vi "Check_Settings_Case.vi"(6 "Queues":T1, 7 "Timer parameters":refnum<vi>, 8 "Status/Errors in":refnum<vi>, 9 "Control Parameters [] in":T2[](array[typedef]) {"Aux Byte Value" format="%02x"; "Max Real Value" format="%#_6e"; "Min Real Value" format="%#_6e"; "dReal/dByte" format="%#_6e"; "Byte Value" format="%02x"; "Identifier" format="%02x"}, 10 "Main parameters in":T5={"Mode"={"Mode"=enum."Dialog", "Expert?"=FALSE, "Dialog?"=FALSE}, "Stop loop"={"Settings changed?"=FALSE, "Stop?"=refnum}, "Send message"={"Send mode"=enum."Get parameters", "Set parameter list"=0, "Get parameter list"=0, "Reset device"=0, "Length set settings message"=0, "Reset buttons?"=FALSE, "Reset Master?"=enum."General"}, "Write settings"={"Options"=enum."File 1"}, "Settings state"={"MAS locked?"=refnum, "SLV locked?"=refnum}, "Button refs"={"Stop program"=refnum, "Save settings"=refnum, "DAQ mode"=refnum, "Reset settings"=refnum, "Apply settings"=refnum, "Reset MAS"=refnum, "Reset SLV"=refnum, "Local DBase?"=refnum, "Last value DBase"=FALSE, "Database"=refnum, "Calibration"=refnum, "Save settings 2"=refnum}, "Update screen"={"Detector number"=0, "Hardware"=enum."None"}, "Files"={"Path config file"=path "", "Path def. ini file"=path "", "Path ini file 1"=path "", "Path ini file 2"=path "", "Path RBF file"=path ""}, "DB connection"={"connection reference"=refnum, "Connected?"=refnum, "ODBC Name"=""}, "Status_id"=refnum, "Time difference"=refnum, "Satellites"=refnum, "Alignment parameters"=refnum, "Page Statistics 2"=refnum, "Database"=refnum, "Page Statistics"=refnum} {"Update screen"."Detector number" format="%#.0f"; "Send message"."Reset device" format="%x"; "Send message"."Get parameter list" format="%x"; "Send message"."Set parameter list" format="%x"}, 11 "Devices in":T4) -> (0 "Status/Errors out":refnum<vi>, 1 "Control Parameters [] out":T2[](array[typedef]) {"Aux Byte Value" format="%02x"; "Max Real Value" format="%#_6e"; "Min Real Value" format="%#_6e"; "dReal/dByte" format="%#_6e"; "Byte Value" format="%02x"; "Identifier" format="%02x"}, 2 "Main parameters out":T5={"Mode"={"Mode"=enum."Dialog", "Expert?"=FALSE, "Dialog?"=FALSE}, "Stop loop"={"Settings changed?"=FALSE, "Stop?"=refnum}, "Send message"={"Send mode"=enum."Get parameters", "Set parameter list"=0, "Get parameter list"=0, "Reset device"=0, "Length set settings message"=0, "Reset buttons?"=FALSE, "Reset Master?"=enum."General"}, "Write settings"={"Options"=enum."File 1"}, "Settings state"={"MAS locked?"=refnum, "SLV locked?"=refnum}, "Button refs"={"Stop program"=refnum, "Save settings"=refnum, "DAQ mode"=refnum, "Reset settings"=refnum, "Apply settings"=refnum, "Reset MAS"=refnum, "Reset SLV"=refnum, "Local DBase?"=refnum, "Last value DBase"=FALSE, "Database"=refnum, "Calibration"=refnum, "Save settings 2"=refnum}, "Update screen"={"Detector number"=0, "Hardware"=enum."None"}, "Files"={"Path config file"=path "", "Path def. ini file"=path "", "Path ini file 1"=path "", "Path ini file 2"=path "", "Path RBF file"=path ""}, "DB connection"={"connection reference"=refnum, "Connected?"=refnum, "ODBC Name"=""}, "Status_id"=refnum, "Time difference"=refnum, "Satellites"=refnum, "Alignment parameters"=refnum, "Page Statistics 2"=refnum, "Database"=refnum, "Page Statistics"=refnum} {"Update screen"."Detector number" format="%#.0f"; "Send message"."Reset device" format="%x"; "Send message"."Get parameter list" format="%x"; "Send message"."Set parameter list" format="%x"}, 3 "Devices out":T4)   [LabVIEW 2013]
uses:
  Controls/Main_Parameters.ctl
  Controls/Mode.ctl
  Controls/Stop_Loop.ctl
  Controls/Send_Message.ctl
  Controls/Send_Message_Mode.ctl
  Controls/Master.ctl
  Controls/Write_Settings.ctl
  Controls/Write_Settings_Options.ctl
  Controls/Settings_State.ctl
  Controls/Button_Refs.ctl
  Controls/Update_Screen.ctl
  Controls/Files.ctl
  Controls/DB_Connection.ctl
  database/Connection.llb/Conn ObjectReference.ctl
  Controls/Devices.ctl
  Controls/Control_Parameters.ctl
  Controls/Queues.ctl
  Controls/One_Second.ctl
  Controls/GPS_Timestamp.ctl
  Controls/Set_Mode.ctl
  Controls/Get_Set_Buttons_mode.ctl
  Controls/Get_Set_Settings_State_Options.ctl
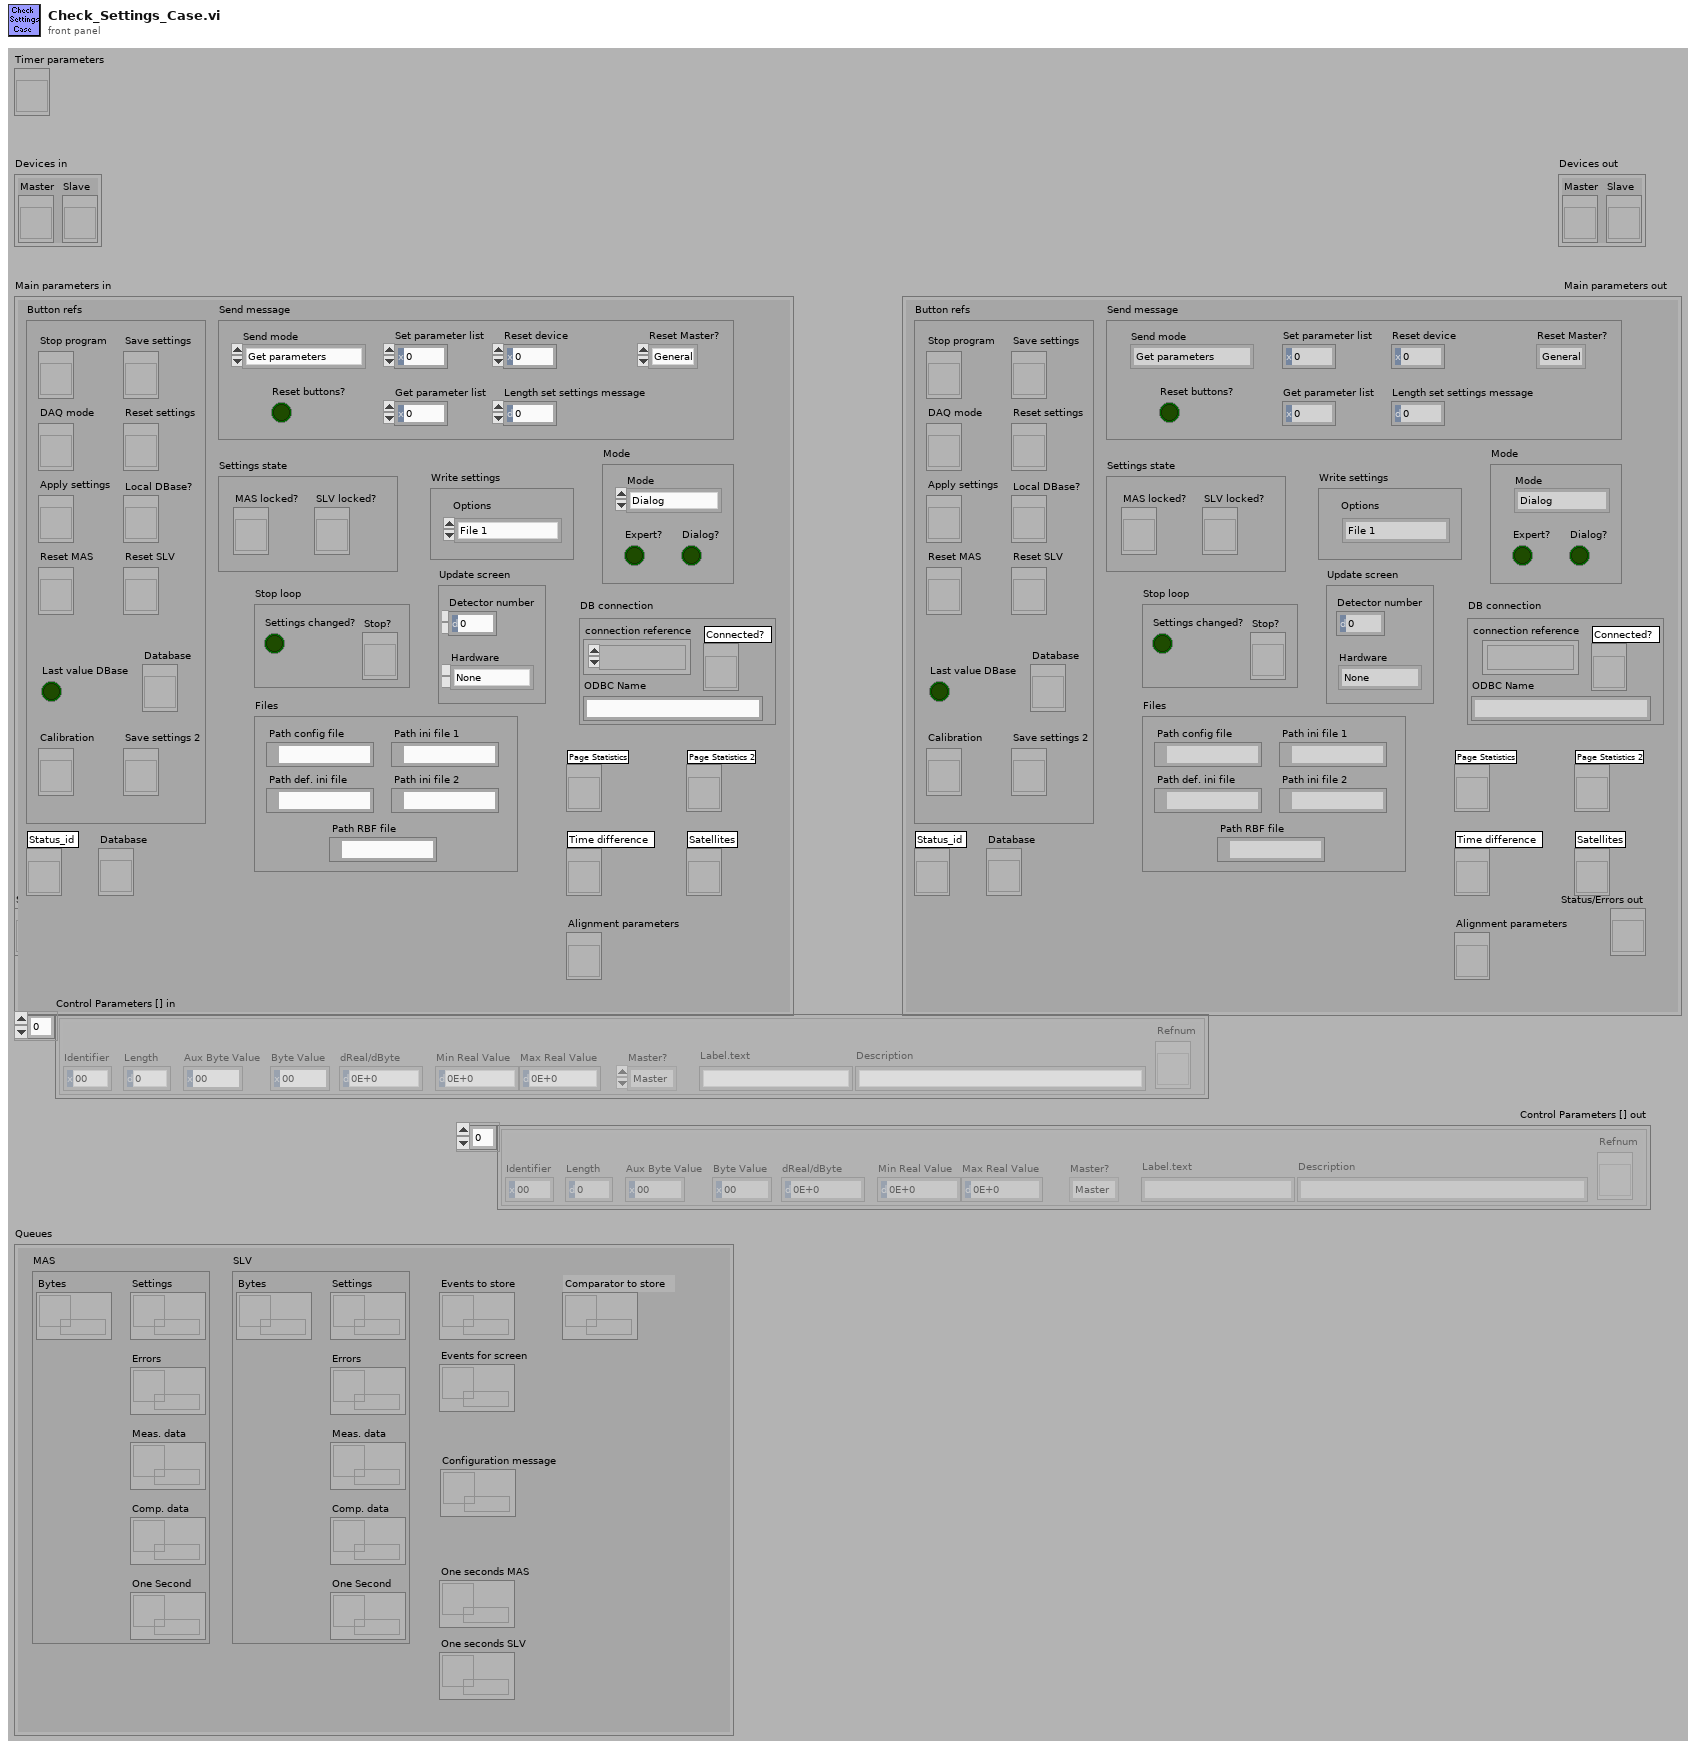
[diagram p1: front panel]
types:
  T1 = typedef "Queues.ctl" = cluster{"MAS":cluster{"Bytes":refnum<queue>, "Settings":refnum<queue>, "Errors":refnum<queue>, "Meas. data":refnum<queue>, "One Second":refnum<queue>, "Comp. data":refnum<queue>}, "SLV":cluster{"Bytes":refnum<queue>, "Settings":refnum<queue>, "Errors":refnum<queue>, "Meas. data":refnum<queue>, "One Second":refnum<queue>, "Comp. data":refnum<queue>}, "Events to store":refnum<queue>, "Events for screen":refnum<queue>, "One seconds MAS":refnum<queue>, "One seconds SLV":refnum<queue>, "Configuration message":refnum<queue>, "Comparator to store":refnum<queue>}
  T2 = typedef "Control_Parameters.ctl" = cluster{"Identifier":u8, "Length":u16, "Byte Value":u32, "dReal/dByte":dbl, "Min Real Value":dbl, "Max Real Value":dbl, "Master?":T3, "Label.text":string, "Description":string, "Refnum":refnum<vi>, "Aux Byte Value":u32}
  T3 = typedef "Master.ctl" = enum16{"Master", "Slave", "General"}
  T4 = typedef "Devices.ctl" = cluster{"Master":refnum<vi>, "Slave":refnum<vi>}
  T5 = typedef "Main_Parameters.ctl" = cluster{"Mode":T6, "Stop loop":T7, "Send message":T8, "Write settings":T10, "Settings state":T12, "Button refs":T13, "Update screen":T14, "Files":T15, "DB connection":T16, "Status_id":refnum<vi>, "Time difference":refnum<vi>, "Satellites":refnum<vi>, "Alignment parameters":refnum<vi>, "Page Statistics 2":refnum<vi>, "Database":refnum<vi>, "Page Statistics":refnum<vi>}
  T6 = typedef "Mode.ctl" = cluster{"Mode":enum8{"Stop", "Dialog", "Hisparc II", "Hisparc II DAQ", "Alignment"}, "Expert?":bool, "Dialog?":bool}
  T7 = typedef "Stop_Loop.ctl" = cluster{"Settings changed?":bool, "Stop?":refnum<vi>}
  T8 = typedef "Send_Message.ctl" = cluster{"Send mode":T9, "Set parameter list":u8, "Get parameter list":u8, "Reset device":u8, "Length set settings message":i32, "Reset buttons?":bool, "Reset Master?":T3}
  T9 = typedef "Send_Message_Mode.ctl" = enum16{"Get parameters", "Set parameters", "From front panel", "From parameters", "Reset device", "Alignment"}
  T10 = typedef "Write_Settings.ctl" = cluster{"Options":T11}
  T11 = typedef "Write_Settings_Options.ctl" = enum16{"File 1", "File 2", "Alignment", "Reset"}
  T12 = typedef "Settings_State.ctl" = cluster{"MAS locked?":refnum<vi>, "SLV locked?":refnum<vi>}
  T13 = typedef "Button_Refs.ctl" = cluster{"Stop program":refnum<vi>, "Save settings":refnum<vi>, "DAQ mode":refnum<vi>, "Reset settings":refnum<vi>, "Apply settings":refnum<vi>, "Reset MAS":refnum<vi>, "Reset SLV":refnum<vi>, "Local DBase?":refnum<vi>, "Last value DBase":bool, "Database":refnum<vi>, "Calibration":refnum<vi>, "Save settings 2":refnum<vi>}
  T14 = typedef "Update_Screen.ctl" = cluster{"Detector number":u16, "Hardware":enum8{"None", "HiSPARC I", "HiSPARC II", "HiSPARC III", "Unknown"}}
  T15 = typedef "Files.ctl" = cluster{"Path config file":path, "Path def. ini file":path, "Path ini file 1":path, "Path ini file 2":path, "Path RBF file":path}
  T16 = typedef "DB_Connection.ctl" = cluster{"connection reference":T17, "Connected?":refnum<vi>, "ODBC Name":string}
  T17 = typedef "Conn ObjectReference.ctl" = refnum<k1>
  T18 = typedef "Set_Mode.ctl" = enum16{"Create Message Only", "Front Panel", "Parameters", "Master", "Slave"}
  T19 = typedef "Settings_Message.ctl" = T20[]
  T20 = typedef "Setting.ctl" = cluster{"Identifier":u8, "  Bytes":u8[], "# Bytes":u16}
  T21 = typedef "Get_Set_Settings_State_Options.ctl" = enum16{"Get", "Lock", "Unlock"}
  T22 = typedef "Get_Set_Buttons_mode.ctl" = enum16{"Get", "Get DAQ", "Set", "Set settings"}
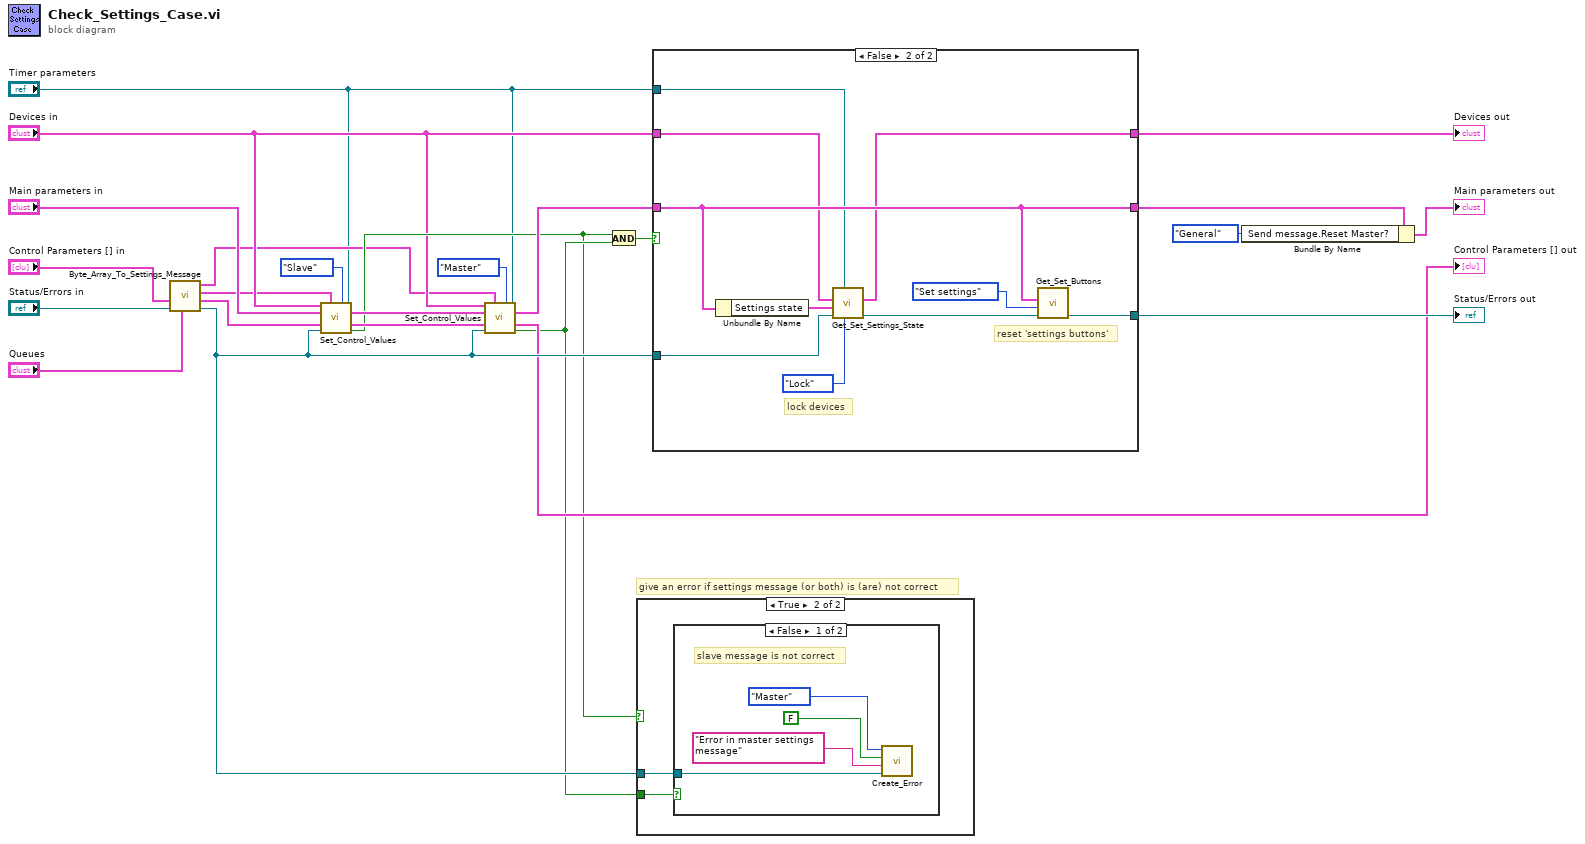
[diagram p0: block diagram]
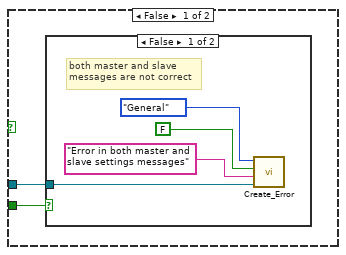
[diagram p2: hidden frame]
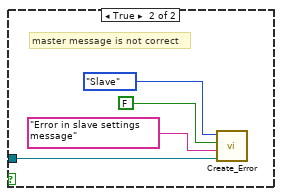
[diagram p3: hidden frame]
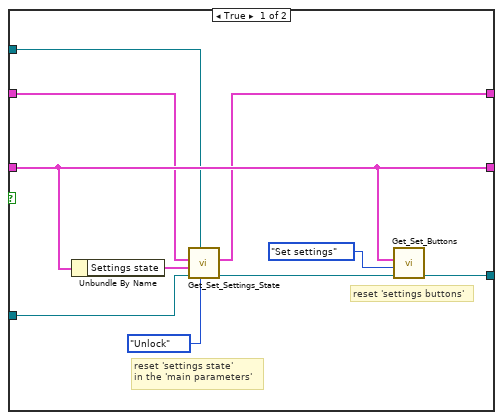
[diagram p5: hidden frame]
diagram:
  # "give an error if settings message (or both) is (are) not correct"
  n1 = call "Byte_Array_To_Settings_Message.vi"("Queues"="Queues", "Status/Errors in"="Status/Errors in", "Control Parameters [] in"="Control Parameters [] in") -> ("Status/Errors out"=w11:refnum<vi>, "Control Parameters [] out"=w18:T2[], "Settings message SLV"=w3:T19, "Settings message MAS"=w2:T19)  [unwired: 5 out]
  n2 = call "Set_Control_Values.vi"("Devices in"="Devices in", "Settings message"=w3, "Set Mode"=Set_Mode."Slave", "Timer parameters in"="Timer parameters", "Main Parameters in"="Main parameters in", "Control Parameters [] in"=w18, "Status/Errors in"=w11) -> ("Main parameters out"=w10:T5, "Control Parameters [] out"=w9:T2[], "Settings ok?"=w5:bool)  [unwired: 6 out]
  n3 = call "Set_Control_Values.vi"("Devices in"="Devices in", "Settings message"=w2, "Set Mode"=Set_Mode."Master", "Timer parameters in"="Timer parameters", "Main Parameters in"=w10, "Control Parameters [] in"=w9, "Status/Errors in"=w11) -> ("Main parameters out"=w8:T5, "Control Parameters [] out"=→"Control Parameters [] out":T2[], "Settings ok?"=w6:bool)  [unwired: 6 out]
  n4 = And(x=w5, y=w6) -> (x .and. y?=w16:bool)
  n5 = case shown="True" w5 {
    tunnel: w11 -> [w25 w35]
    tunnel: w6 -> [w26 w36]
    frame False {
      n6 = case shown="False" w26 {
        tunnel: w25 -> [w27 w31]
        frame False {
          # "both master and slave\nmessages are not correct"
          n7 = call "Create_Error.vi"("Status/Errors in"=w27, "HiSPARC error"="Error in both master and slave settings messages", "Warning? (false)"=FALSE, "Master?"=Master."General") -> ()  [unwired: 2 in, 6 out]
        }
        frame True {
          # "master message is not correct"
          n8 = call "Create_Error.vi"("Status/Errors in"=w31, "HiSPARC error"="Error in slave settings message", "Warning? (false)"=FALSE, "Master?"=Master."Slave") -> ()  [unwired: 2 in, 6 out]
        }
      }
    }
    frame True {
      n9 = case shown="False" w36 {
        tunnel: w35 -> [w37 _]
        frame False {
          # "slave message is not correct"
          n10 = call "Create_Error.vi"("Status/Errors in"=w37, "HiSPARC error"="Error in master settings message", "Warning? (false)"=FALSE, "Master?"=Master."Master") -> ()  [unwired: 2 in, 6 out]
        }
        frame True {
          # "both master and slave messages correct"
        }
      }
    }
  }
  n11 = case shown="False" w16 {
    tunnel: [w47 w57] -> w24
    tunnel: w8 -> [w45 w55]
    tunnel: [w45 w55] -> w13
    tunnel: w11 -> [w44 w54]
    tunnel: "Timer parameters" -> [w43 w53]
    tunnel: "Devices in" -> [w42 w52]
    tunnel: [w41 w51] -> w15
    frame True {
      # "reset 'settings state'\nin the 'main parameters'"
      # "reset 'settings buttons'"
      n12 = Unbundle By Name(w45) -> ("Settings state"=w50:T12)
      n13 = call "Get_Set_Settings_State.vi"("Get/Set"=Get_Set_Settings_State_Options."Unlock", "Timer parameters"=w43, "Status/Errors in"=w44, "Settings state"=w50, "Devices in"=w42) -> ("Status/Errors out"=w49:refnum<vi>, "Devices out"=w41:T4)  [unwired: 5 out]
      n14 = call "Get_Set_Buttons.vi"("Status/Errors in"=w49, "Set?"=Get_Set_Buttons_mode."Set settings", "Main parameters"=w45) -> ("Status/Errors out"=w47:refnum<vi>)  [unwired: 8 out]
    }
    frame False {
      # "lock devices"
      # "reset 'settings buttons'"
      n15 = Unbundle By Name(w55) -> ("Settings state"=w60:T12)
      n16 = call "Get_Set_Settings_State.vi"("Get/Set"=Get_Set_Settings_State_Options."Lock", "Timer parameters"=w53, "Status/Errors in"=w54, "Settings state"=w60, "Devices in"=w52) -> ("Status/Errors out"=w59:refnum<vi>, "Devices out"=w51:T4)  [unwired: 5 out]
      n17 = call "Get_Set_Buttons.vi"("Status/Errors in"=w59, "Set?"=Get_Set_Buttons_mode."Set settings", "Main parameters"=w55) -> ("Status/Errors out"=w57:refnum<vi>)  [unwired: 8 out]
    }
  }
  "Devices out" <- w15
  "Status/Errors out" <- w24
  n18 = Bundle By Name(cluster=w13, "Send message.Reset Master?"=Master."General") -> (→"Main parameters out":T5)
